vi "ATF Storage-CDT Target FGV.vi"(7 "Enum":enum16{"Write", "Read", "Init"}(ring)=enum."Read", 8 "error in":errorcluster, 9 "Time Stamp":timestamp) -> (0 "error out":errorcluster, 1 "Time StampOut":timestamp)   [LabVIEW 2022 SP3]
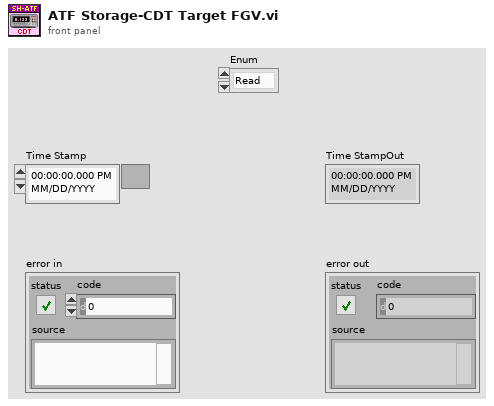
[diagram p1: front panel]
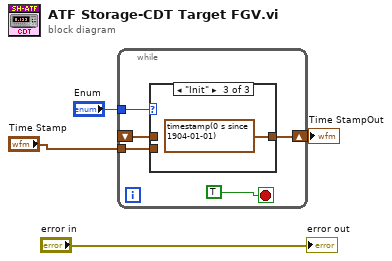
[diagram p0: block diagram]
diagram:
  n1 = while {
    tunnel: "Enum" -> [w9]
    tunnel: "Time Stamp" -> [w7]
    shift-right: [w6] -> w1
    shift-left: _ -> [w5]
    stop <- TRUE stop-if-true
    n2 = case shown="\"Init\"" w9 {
      tunnel: w7 -> [w10 _ _]
      tunnel: [w10 w11 timestamp(0 s since 1904-01-01) ("Time Stamp")] -> w6
      tunnel: w5 -> [_ w11 _]
      frame "Write", Default {
      }
      frame "Read" {
      }
      frame "Init" {
      }
    }
  }
  "Time StampOut" <- w1
  "error out" <- "error in"
